vi "Begin.vi"(11 "Image Size":T1=enum."160x120") -> (0 "error out":errorcluster)   [LabVIEW 2012]
doc: "Called before other user functions, this VI is expected to open initial I/O refnums, load in file data, and do all program initialization. Notice that the <B>error out</B> terminal is simply used for data flow. Wiring it to other structures or subVIs ensures that this VI runs first."
uses:
  <vilib>/Rock Robotics/WPI/Camera/WPI_CameraImageSize.ctl
  <vilib>/Rock Robotics/WPI/Camera/WPI_CameraWhite Balance Values.ctl
  <vilib>/Rock Robotics/WPI/Camera/WPI_CameraExposure Values.ctl
  <vilib>/Rock Robotics/WPI/Camera/WPI_CameraFrameRate.ctl
  <vilib>/Rock Robotics/WPI/DriverStation/WPI_DriverStationRobotMode2.ctl
  <vilib>/Rock Robotics/WPI/Joystick/WPI_JoystickDeviceEnum.ctl
  <vilib>/Rock Robotics/WPI/CAN/Jaguar/SubVIs/WPI_CANJaguar_ControlMode.ctl
  <vilib>/Rock Robotics/WPI/CAN/Jaguar/SubVIs/WPI_CANJaguar_PositionReference.ctl
  <vilib>/Rock Robotics/WPI/CAN/Jaguar/SubVIs/WPI_CANJaguar_SpeedReference.ctl
  Robot Global Data.vi
  <vilib>/Rock Robotics/WPI/MotorControl/WPI_MotorControlOpenCANJaguar.vi
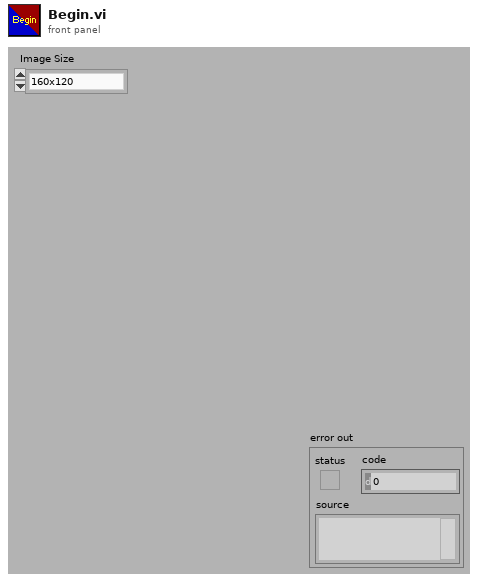
[diagram p1: front panel]
types:
  T1 = typedef "WPI_CameraImageSize.ctl" = enum16{"640x480", "320x240", "160x120"}
  T2 = typedef "WPI_CANJaguar_SpeedReference.ctl" = u8
  T3 = typedef "WPI_CANJaguar_ControlMode.ctl" = enum8{"Percent VBus", "Current", "Speed", "Position", "Voltage"}
  T4 = typedef "WPI_CANJaguar_PositionReference.ctl" = u8
  T5 = typedef "WPI_JoystickDeviceEnum.ctl" = enum16{"USB 1", "USB 2", "USB 3", "USB 4", "Kinect 1", "Kinect 2"}
  T6 = typedef "WPI_DriverStationRobotMode2.ctl" = enum16{"Autonomous Disabled", "Autonomous Enabled", "Teleop Disabled", "Teleop Enabled", "Timeout", "Finish", "Test Disabled", "Test Enabled"}
  T7 = typedef "WPI_CameraFrameRate.ctl" = u32
  T8 = typedef "WPI_CameraExposure Values.ctl" = enum16{"Auto", "Flicker-free 50 Hz", "Flicker-free 60 Hz", "Hold current"}
  T9 = typedef "WPI_CameraWhite Balance Values.ctl" = enum16{"Auto", "Fixed indoor", "Fixed outdoor 1", "Fixed outdoor 2", "Fixed fluorescent 1", "Fixed fluorescent 2", "Hold current"}
  T10 = typedef "WPI_JoystickDevRef.ctl" = cluster{"Device":T5}
  T11 = typedef "WPI_CameraDevRef.ctl" = cluster{"Camera Address":string, "CameraStatus":errorcluster, "Acquire Image Notifier":refnum<notifier>}
  T12 = typedef "WPI_MotorControlDeviceRef.ctl" = cluster{"DeviceStatus":errorcluster, "Type":enum16{"PWM", "CAN"}, "PWM":cluster{"Digital Module":T13, "PWM Channel":T14, "DeadBand":T15}, "CAN":cluster{"Device Number":u8, "Control Mode":T3, "Semaphore":T16, "Max Vout":dbl}, "Invert":bool, "TransformRef":T17, "InvTransformRef":T17}
  T13 = typedef "FPGA_TypedefDigitalModule.ctl" = enum16{"Digital Module 1", "Digital Module 2"}
  T14 = typedef "FPGA_DIOPWMChannel.ctl" = enum8{"PWM 1", "PWM 2", "PWM 3", "PWM 4", "PWM 5", "PWM 6", "PWM 7", "PWM 8", "PWM 9", "PWM 10", "Invalid"}
  T15 = typedef "WPI_PWMDeadband.ctl" = cluster{"Name":string, "maxPositivePwm":i32, "minPositivePwm":i32, "centerPwm":i32, "maxNegativePwm":i32, "minNegativePwm":i32, "angularRange":u16}
  T16 = typedef "Semaphore RefNum" = refnum<k1>
  T17 = typedef "WPI_PWMTransform_ConPane.ctl" = refnum<vi>
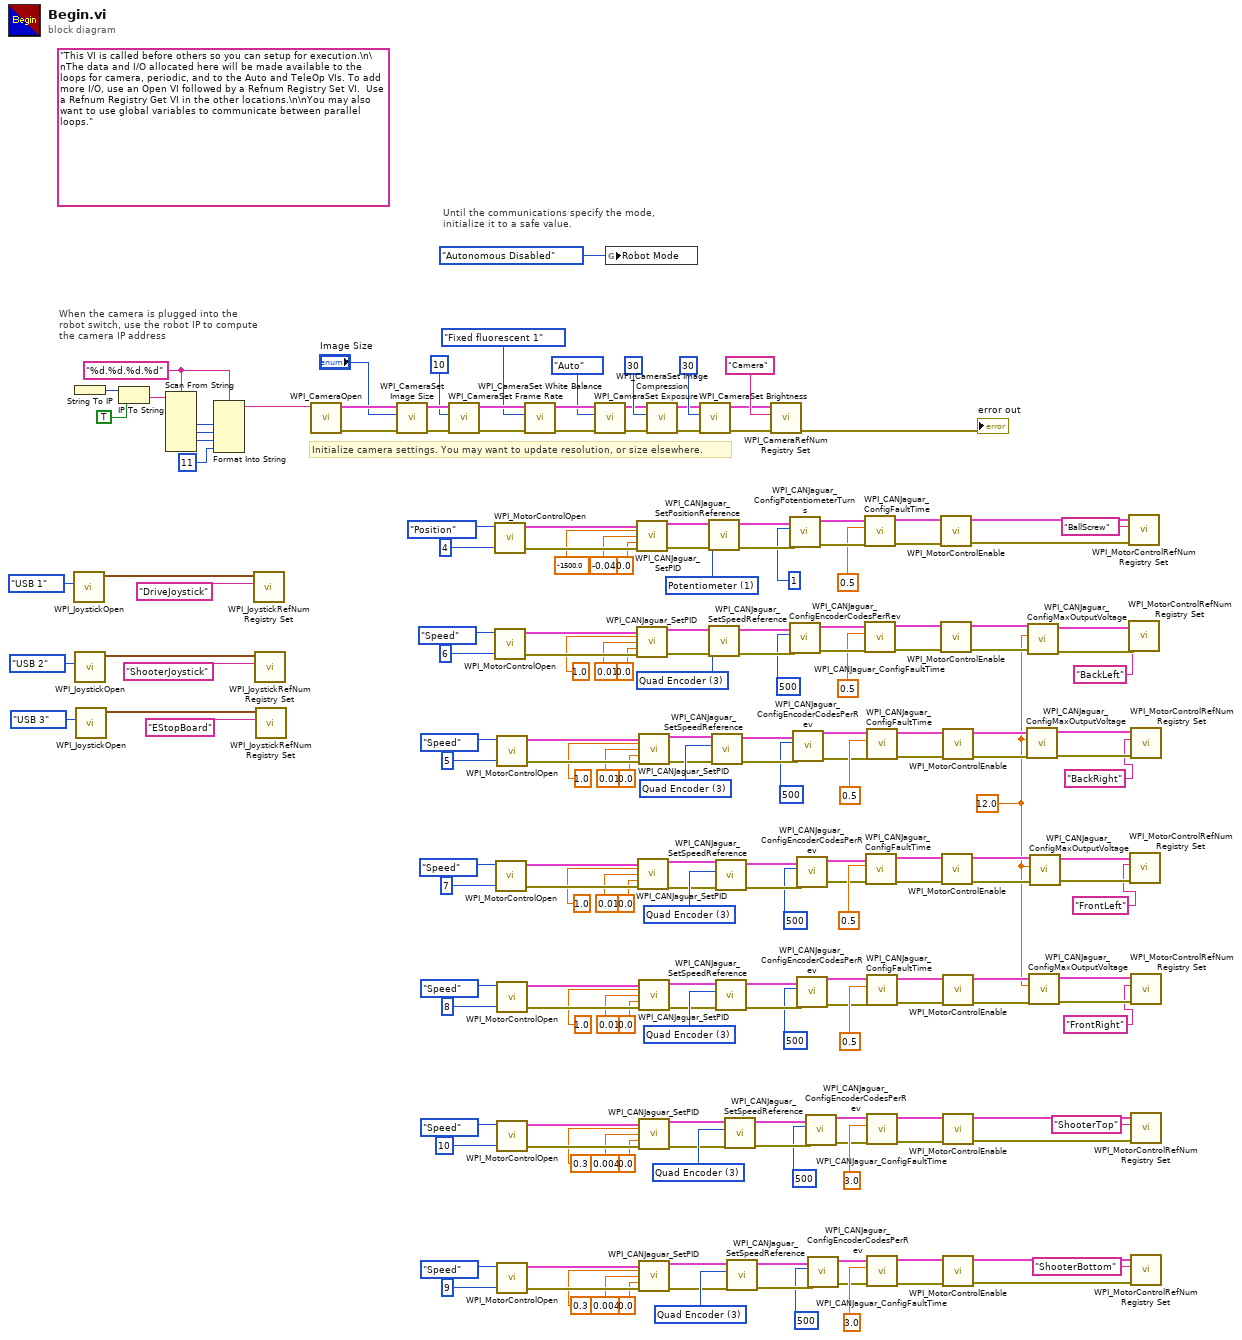
[diagram p0: block diagram]
diagram:
  w23 = T2 3 items=["Encoder"=0, "Inv Encoder"=2, "Quad Encoder"=3, "None"=255] ("Speed Reference")
  w27 = T2 3 items=["Encoder"=0, "Inv Encoder"=2, "Quad Encoder"=3, "None"=255] ("Speed Reference")
  w31 = T2 3 items=["Encoder"=0, "Inv Encoder"=2, "Quad Encoder"=3, "None"=255] ("Speed Reference")
  w35 = T2 3 items=["Encoder"=0, "Inv Encoder"=2, "Quad Encoder"=3, "None"=255] ("Speed Reference")
  w39 = T2 3 items=["Encoder"=0, "Inv Encoder"=2, "Quad Encoder"=3, "None"=255] ("Speed Reference")
  w43 = 12.0 ("Fault Time (s)")
  w64 = T2 3 items=["Encoder"=0, "Inv Encoder"=2, "Quad Encoder"=3, "None"=255] ("Speed Reference")
  w147 = T4 1 items=["Quad Encoder"=0, "Potentiometer"=1, "None"=255] ("Position Reference")
  w169 = "%d.%d.%d.%d" ("format string")
  (unwired) "This VI is called before others so you can setup for execution.\n\nThe data and I/O allocated here will be made available to the loops for camera, periodic, and to the Auto and TeleOp VIs. To add more I/O, use an Open VI followed by a Refnum Registry Set VI.  Use a Refnum Registry Get VI in the other locations.\n\nYou may also want to use global variables to communicate between parallel loops."
  # "Until the communications specify the mode,\ninitialize it to a safe value."
  # "When the camera is plugged into the\nrobot switch, use the robot IP to compute\nthe camera IP address"
  # "Initialize camera settings. You may want to update resolution, or size elsewhere."
  n1 = call <vilib>:"WPI_JoystickOpen.vi"("JoystickDevice"=WPI_JoystickDeviceEnum."USB 1") -> ("JoystickDevRef"=w165:T10)  [unwired: 10 in]
  n2 = String To IP() -> (0:w176:u32)  [unwired: 1 in]
  n3 = call <vilib>:"WPI_JoystickOpen.vi"("JoystickDevice"=WPI_JoystickDeviceEnum."USB 2") -> ("JoystickDevRef"=w161:T10)  [unwired: 10 in]
  n4 = call <vilib>:"WPI_JoystickOpen.vi"("JoystickDevice"=WPI_JoystickDeviceEnum."USB 3") -> ("JoystickDevRef"=w158:T10)  [unwired: 10 in]
  n5 = IP To String(1:TRUE ("dot notation? (F)"), 2:w176) -> (0:w174:string)
  n6 = Scan From String(format string=w169, input string=w174) -> (output 1=w173:i32, output 2=w172:i32, output 3=w171:i32)  [unwired: 7 in, 3 out]
  n7 = Format Into String(format string=w169, w173, w172, w171, 11 ("Compression")) -> (resulting string=w167:string)  [unwired: 2 in, 1 out]
  n8 = call <vilib>:"WPI_JoystickRefNum Registry Set.vi"("refnum name"="DriveJoystick", "JoystickDevRef"=w165) -> ()  [unwired: 8 in, 2 out]
  n9 = call <vilib>:"WPI_JoystickRefNum Registry Set.vi"("refnum name"="ShooterJoystick", "JoystickDevRef"=w161) -> ()  [unwired: 8 in, 2 out]
  n10 = call <vilib>:"WPI_JoystickRefNum Registry Set.vi"("refnum name"="EStopBoard", "JoystickDevRef"=w158) -> ()  [unwired: 8 in, 2 out]
  n11 = call <vilib>:"WPI_CameraOpen.vi"("Camera Address"=w167) -> ("error out"=w188:errorcluster, "CameraDevRef"=w189:T11)  [unwired: 1 in, 8 out]
  n12 = call <vilib>:"WPI_CameraSet Image Size.vi"("error in (no error)"=w188, "Image Size"="Image Size", "CameraDevRef"=w189) -> ("error out"=w187:errorcluster, "CameraDevRef Out"=w190:T11)  [unwired: 7 out]
  n13 = call <vilib>:"WPI_CameraSet Frame Rate.vi"("error in (no error)"=w187, "Frame Rate (fps)"=T7 10, "CameraDevRef"=w190) -> ("error out"=w186:errorcluster, "CameraDevRef Out"=w192:T11)  [unwired: 7 out]
  n14 = call-poly <vilib>:"WPI_MotorControlOpen.vi"("Device Number"=u8 4, "Control Mode"=WPI_CANJaguar_ControlMode."Position") -> ("error out"=w153:errorcluster, "MotorControlDeviceRef"=w154:T12)  [unwired: 8 in]
  n15 = call-poly <vilib>:"WPI_MotorControlOpen.vi"("Device Number"=u8 6, "Control Mode"=WPI_CANJaguar_ControlMode."Speed") -> ("error out"=w133:errorcluster, "MotorControlDeviceRef"=w134:T12)  [unwired: 8 in]
  n16 = call-poly <vilib>:"WPI_MotorControlOpen.vi"("Device Number"=u8 7, "Control Mode"=WPI_CANJaguar_ControlMode."Speed") -> ("error out"=w106:errorcluster, "MotorControlDeviceRef"=w107:T12)  [unwired: 8 in]
  n17 = call-poly <vilib>:"WPI_MotorControlOpen.vi"("Device Number"=u8 5, "Control Mode"=WPI_CANJaguar_ControlMode."Speed") -> ("error out"=w116:errorcluster, "MotorControlDeviceRef"=w117:T12)  [unwired: 8 in]
  n18 = call-poly <vilib>:"WPI_MotorControlOpen.vi"("Device Number"=u8 8, "Control Mode"=WPI_CANJaguar_ControlMode."Speed") -> ("error out"=w96:errorcluster, "MotorControlDeviceRef"=w97:T12)  [unwired: 8 in]
  n19 = call-poly <vilib>:"WPI_MotorControlOpen.vi"("Device Number"=u8 10, "Control Mode"=WPI_CANJaguar_ControlMode."Speed") -> ("error out"=w86:errorcluster, "MotorControlDeviceRef"=w87:T12)  [unwired: 8 in]
  n20 = call-poly <vilib>:"WPI_MotorControlOpen.vi"("Device Number"=u8 9, "Control Mode"=WPI_CANJaguar_ControlMode."Speed") -> ("error out"=w74:errorcluster, "MotorControlDeviceRef"=w75:T12)  [unwired: 8 in]
  n21 = call <vilib>:"WPI_CameraSet White Balance.vi"("error in (no error)"=w186, "White Balance"=WPI_CameraWhite_Balance_Values."Fixed fluorescent 1", "CameraDevRef"=w192) -> ("error out"=w185:errorcluster, "CameraDevRef Out"=w191:T11)  [unwired: 7 out]
  n22 = call <vilib>:"WPI_CameraSet Exposure.vi"("error in (no error)"=w185, "Exposure"=WPI_CameraExposure_Values."Auto", "CameraDevRef"=w191) -> ("error out"=w184:errorcluster, "CameraDevRef Out"=w194:T11)  [unwired: 7 out]
  n23 = global write "Robot Global Data.vi" "Robot Mode"(WPI_DriverStationRobotMode2."Autonomous Disabled" ("Robot Mode")) -> ()
  n24 = call <vilib>:"WPI_CANJaguar_SetPID.vi"("CAN Jaguar Ref"=w154, "P"=-1500.0, "I"=-0.04, "D"=0.0, "error in (no error)"=w153) -> ("CAN Jaguar Ref Out"=w149:T12, "error out"=w148:errorcluster)  [unwired: 9 in]
  n25 = call <vilib>:"WPI_CANJaguar_SetPID.vi"("CAN Jaguar Ref"=w134, "P"=1.0, "I"=0.01, "D"=0.0, "error in (no error)"=w133) -> ("CAN Jaguar Ref Out"=w129:T12, "error out"=w128:errorcluster)  [unwired: 9 in]
  n26 = call <vilib>:"WPI_CANJaguar_SetPID.vi"("CAN Jaguar Ref"=w107, "P"=1.0, "I"=0.01, "D"=0.0, "error in (no error)"=w106) -> ("CAN Jaguar Ref Out"=w6:T12, "error out"=w5:errorcluster)  [unwired: 9 in]
  n27 = call <vilib>:"WPI_CANJaguar_SetPID.vi"("CAN Jaguar Ref"=w117, "P"=1.0, "I"=0.01, "D"=0.0, "error in (no error)"=w116) -> ("CAN Jaguar Ref Out"=w10:T12, "error out"=w9:errorcluster)  [unwired: 9 in]
  n28 = call <vilib>:"WPI_CANJaguar_SetPID.vi"("CAN Jaguar Ref"=w97, "P"=1.0, "I"=0.01, "D"=0.0, "error in (no error)"=w96) -> ("CAN Jaguar Ref Out"=w13:T12, "error out"=w14:errorcluster)  [unwired: 9 in]
  n29 = call <vilib>:"WPI_CANJaguar_SetPID.vi"("CAN Jaguar Ref"=w87, "P"=0.3, "I"=0.004, "D"=0.0, "error in (no error)"=w86) -> ("CAN Jaguar Ref Out"=w15:T12, "error out"=w16:errorcluster)  [unwired: 9 in]
  n30 = call <vilib>:"WPI_CANJaguar_SetPID.vi"("CAN Jaguar Ref"=w75, "P"=0.3, "I"=0.004, "D"=0.0, "error in (no error)"=w74) -> ("CAN Jaguar Ref Out"=w22:T12, "error out"=w21:errorcluster)  [unwired: 9 in]
  n31 = call <vilib>:"WPI_CameraSet Image Compression.vi"("error in (no error)"=w184, "Compression"=30, "CameraDevRef"=w194) -> ("error out"=w183:errorcluster, "CameraDevRef Out"=w193:T11)  [unwired: 7 out]
  n32 = call <vilib>:"WPI_CameraSet Brightness.vi"("error in (no error)"=w183, "Brightness"=30, "CameraDevRef"=w193) -> ("error out"=w181:errorcluster, "CameraDevRef Out"=w182:T11)  [unwired: 7 out]
  n33 = call <vilib>:"WPI_CANJaguar_SetPositionReference.vi"("error in (no error)"=w148, "Position Reference"=w147, "CAN Jaguar Ref"=w149) -> ("error out"=w145:errorcluster, "CAN Jaguar Ref Out"=w146:T12)  [unwired: 7 in]
  n34 = call <vilib>:"WPI_CANJaguar_SetSpeedReference.vi"("error in (no error)"=w128, "Speed Reference"=w64, "CAN Jaguar Ref"=w129) -> ("error out"=w126:errorcluster, "CAN Jaguar Ref Out"=w127:T12)  [unwired: 7 in]
  n35 = call <vilib>:"WPI_CANJaguar_SetSpeedReference.vi"("error in (no error)"=w9, "Speed Reference"=w39, "CAN Jaguar Ref"=w10) -> ("error out"=w41:errorcluster, "CAN Jaguar Ref Out"=w42:T12)  [unwired: 7 in]
  n36 = call <vilib>:"WPI_CANJaguar_SetSpeedReference.vi"("error in (no error)"=w5, "Speed Reference"=w35, "CAN Jaguar Ref"=w6) -> ("error out"=w37:errorcluster, "CAN Jaguar Ref Out"=w38:T12)  [unwired: 7 in]
  n37 = call <vilib>:"WPI_CANJaguar_SetSpeedReference.vi"("error in (no error)"=w14, "Speed Reference"=w31, "CAN Jaguar Ref"=w13) -> ("error out"=w33:errorcluster, "CAN Jaguar Ref Out"=w34:T12)  [unwired: 7 in]
  n38 = call <vilib>:"WPI_CANJaguar_SetSpeedReference.vi"("error in (no error)"=w16, "Speed Reference"=w27, "CAN Jaguar Ref"=w15) -> ("error out"=w29:errorcluster, "CAN Jaguar Ref Out"=w30:T12)  [unwired: 7 in]
  n39 = call <vilib>:"WPI_CANJaguar_SetSpeedReference.vi"("error in (no error)"=w21, "Speed Reference"=w23, "CAN Jaguar Ref"=w22) -> ("error out"=w25:errorcluster, "CAN Jaguar Ref Out"=w26:T12)  [unwired: 7 in]
  n40 = call <vilib>:"WPI_CameraRefNum Registry Set.vi"("error in (no error)"=w181, "refnum name"="Camera", "CameraDevRef"=w182) -> ("error out"=→"error out":errorcluster)  [unwired: 8 out]
  n41 = call <vilib>:"WPI_CANJaguar_ConfigPotentiometerTurns.vi"("error in (no error)"=w145, "Potentiometer Turns"=u16 1, "CAN Jaguar Ref"=w146) -> ("error out"=w142:errorcluster, "CAN Jaguar Ref Out"=w143:T12)  [unwired: 7 in]
  n42 = call <vilib>:"WPI_CANJaguar_ConfigEncoderCodesPerRev.vi"("error in (no error)"=w126, "Encoder Codes Per Rev"=u16 500 ("Potentiometer Turns"), "CAN Jaguar Ref"=w127) -> ("error out"=w123:errorcluster, "CAN Jaguar Ref Out"=w124:T12)  [unwired: 7 in]
  n43 = call <vilib>:"WPI_CANJaguar_ConfigEncoderCodesPerRev.vi"("error in (no error)"=w41, "Encoder Codes Per Rev"=u16 500 ("Potentiometer Turns"), "CAN Jaguar Ref"=w42) -> ("error out"=w8:errorcluster, "CAN Jaguar Ref Out"=w7:T12)  [unwired: 7 in]
  n44 = call <vilib>:"WPI_CANJaguar_ConfigEncoderCodesPerRev.vi"("error in (no error)"=w37, "Encoder Codes Per Rev"=u16 500 ("Potentiometer Turns"), "CAN Jaguar Ref"=w38) -> ("error out"=w3:errorcluster, "CAN Jaguar Ref Out"=w4:T12)  [unwired: 7 in]
  n45 = call <vilib>:"WPI_CANJaguar_ConfigEncoderCodesPerRev.vi"("error in (no error)"=w33, "Encoder Codes Per Rev"=u16 500 ("Potentiometer Turns"), "CAN Jaguar Ref"=w34) -> ("error out"=w12:errorcluster, "CAN Jaguar Ref Out"=w11:T12)  [unwired: 7 in]
  n46 = call <vilib>:"WPI_CANJaguar_ConfigEncoderCodesPerRev.vi"("error in (no error)"=w29, "Encoder Codes Per Rev"=u16 500 ("Potentiometer Turns"), "CAN Jaguar Ref"=w30) -> ("error out"=w18:errorcluster, "CAN Jaguar Ref Out"=w17:T12)  [unwired: 7 in]
  n47 = call <vilib>:"WPI_CANJaguar_ConfigEncoderCodesPerRev.vi"("error in (no error)"=w25, "Encoder Codes Per Rev"=u16 500 ("Potentiometer Turns"), "CAN Jaguar Ref"=w26) -> ("error out"=w19:errorcluster, "CAN Jaguar Ref Out"=w20:T12)  [unwired: 7 in]
  n48 = call <vilib>:"WPI_CANJaguar_ConfigFaultTime.vi"("error in (no error)"=w142, "Fault Time (s)"=0.5, "CAN Jaguar Ref"=w143) -> ("error out"=w139:errorcluster, "CAN Jaguar Ref Out"=w140:T12)  [unwired: 7 in]
  n49 = call <vilib>:"WPI_CANJaguar_ConfigFaultTime.vi"("error in (no error)"=w123, "Fault Time (s)"=0.5, "CAN Jaguar Ref"=w124) -> ("error out"=w120:errorcluster, "CAN Jaguar Ref Out"=w121:T12)  [unwired: 7 in]
  n50 = call <vilib>:"WPI_CANJaguar_ConfigFaultTime.vi"("error in (no error)"=w3, "Fault Time (s)"=0.5, "CAN Jaguar Ref"=w4) -> ("error out"=w100:errorcluster, "CAN Jaguar Ref Out"=w101:T12)  [unwired: 7 in]
  n51 = call <vilib>:"WPI_CANJaguar_ConfigFaultTime.vi"("error in (no error)"=w8, "Fault Time (s)"=0.5, "CAN Jaguar Ref"=w7) -> ("error out"=w110:errorcluster, "CAN Jaguar Ref Out"=w111:T12)  [unwired: 7 in]
  n52 = call <vilib>:"WPI_CANJaguar_ConfigFaultTime.vi"("error in (no error)"=w12, "Fault Time (s)"=0.5, "CAN Jaguar Ref"=w11) -> ("error out"=w90:errorcluster, "CAN Jaguar Ref Out"=w91:T12)  [unwired: 7 in]
  n53 = call <vilib>:"WPI_CANJaguar_ConfigFaultTime.vi"("error in (no error)"=w18, "Fault Time (s)"=3.0, "CAN Jaguar Ref"=w17) -> ("error out"=w80:errorcluster, "CAN Jaguar Ref Out"=w81:T12)  [unwired: 7 in]
  n54 = call <vilib>:"WPI_CANJaguar_ConfigFaultTime.vi"("error in (no error)"=w19, "Fault Time (s)"=3.0, "CAN Jaguar Ref"=w20) -> ("error out"=w68:errorcluster, "CAN Jaguar Ref Out"=w69:T12)  [unwired: 7 in]
  n55 = call <vilib>:"WPI_MotorControlEnable.vi"("error in (no error)"=w139, "CAN Jaguar Ref"=w140) -> ("error out"=w137:errorcluster, "CAN Jaguar Ref Out"=w138:T12)  [unwired: 8 in]
  n56 = call <vilib>:"WPI_MotorControlEnable.vi"("error in (no error)"=w120, "CAN Jaguar Ref"=w121) -> ("error out"=w62:errorcluster, "CAN Jaguar Ref Out"=w63:T12)  [unwired: 8 in]
  n57 = call <vilib>:"WPI_MotorControlEnable.vi"("error in (no error)"=w100, "CAN Jaguar Ref"=w101) -> ("error out"=w50:errorcluster, "CAN Jaguar Ref Out"=w51:T12)  [unwired: 8 in]
  n58 = call <vilib>:"WPI_MotorControlEnable.vi"("error in (no error)"=w110, "CAN Jaguar Ref"=w111) -> ("error out"=w57:errorcluster, "CAN Jaguar Ref Out"=w58:T12)  [unwired: 8 in]
  n59 = call <vilib>:"WPI_MotorControlEnable.vi"("error in (no error)"=w90, "CAN Jaguar Ref"=w91) -> ("error out"=w47:errorcluster, "CAN Jaguar Ref Out"=w48:T12)  [unwired: 8 in]
  n60 = call <vilib>:"WPI_MotorControlEnable.vi"("error in (no error)"=w80, "CAN Jaguar Ref"=w81) -> ("error out"=w78:errorcluster, "CAN Jaguar Ref Out"=w79:T12)  [unwired: 8 in]
  n61 = call <vilib>:"WPI_MotorControlEnable.vi"("error in (no error)"=w68, "CAN Jaguar Ref"=w69) -> ("error out"=w66:errorcluster, "CAN Jaguar Ref Out"=w67:T12)  [unwired: 8 in]
  n62 = call <vilib>:"WPI_CANJaguar_ConfigMaxOutputVoltage.vi"("error in (no error)"=w57, "Maximum Output Voltage"=w43, "CAN Jaguar Ref"=w58) -> ("error out"=w56:errorcluster, "CAN Jaguar Ref Out"=w55:T12)  [unwired: 7 in]
  n63 = call <vilib>:"WPI_CANJaguar_ConfigMaxOutputVoltage.vi"("error in (no error)"=w62, "Maximum Output Voltage"=w43, "CAN Jaguar Ref"=w63) -> ("error out"=w61:errorcluster, "CAN Jaguar Ref Out"=w60:T12)  [unwired: 7 in]
  n64 = call <vilib>:"WPI_CANJaguar_ConfigMaxOutputVoltage.vi"("error in (no error)"=w47, "Maximum Output Voltage"=w43, "CAN Jaguar Ref"=w48) -> ("error out"=w45:errorcluster, "CAN Jaguar Ref Out"=w46:T12)  [unwired: 7 in]
  n65 = call <vilib>:"WPI_CANJaguar_ConfigMaxOutputVoltage.vi"("error in (no error)"=w50, "Maximum Output Voltage"=w43, "CAN Jaguar Ref"=w51) -> ("error out"=w52:errorcluster, "CAN Jaguar Ref Out"=w53:T12)  [unwired: 7 in]
  n66 = call <vilib>:"WPI_MotorControlRefNum Registry Set.vi"("error in (no error)"=w137, "refnum name"="BallScrew", "MotorControlDevRef"=w138) -> ()  [unwired: 7 in, 2 out]
  n67 = call <vilib>:"WPI_MotorControlRefNum Registry Set.vi"("error in (no error)"=w61, "refnum name"="BackLeft", "MotorControlDevRef"=w60) -> ()  [unwired: 7 in, 2 out]
  n68 = call <vilib>:"WPI_MotorControlRefNum Registry Set.vi"("error in (no error)"=w52, "refnum name"="FrontLeft", "MotorControlDevRef"=w53) -> ()  [unwired: 7 in, 2 out]
  n69 = call <vilib>:"WPI_MotorControlRefNum Registry Set.vi"("error in (no error)"=w56, "refnum name"="BackRight", "MotorControlDevRef"=w55) -> ()  [unwired: 7 in, 2 out]
  n70 = call <vilib>:"WPI_MotorControlRefNum Registry Set.vi"("error in (no error)"=w45, "refnum name"="FrontRight", "MotorControlDevRef"=w46) -> ()  [unwired: 7 in, 2 out]
  n71 = call <vilib>:"WPI_MotorControlRefNum Registry Set.vi"("error in (no error)"=w78, "refnum name"="ShooterTop", "MotorControlDevRef"=w79) -> ()  [unwired: 7 in, 2 out]
  n72 = call <vilib>:"WPI_MotorControlRefNum Registry Set.vi"("error in (no error)"=w66, "refnum name"="ShooterBottom", "MotorControlDevRef"=w67) -> ()  [unwired: 7 in, 2 out]
